vi "Instantiate.vi"(0 "location":string, 5 "insecurePort":string, 11 "error in (no error)":errorcluster) -> (4 "Measurement Client Wrapper out":refnum<class "Measurement Client Wrapper.lvclass">, 15 "error out":errorcluster)   [LabVIEW 2020, in "Measurement Client Wrapper.lvclass"]
uses:
  Measurement Client Wrapper.lvclass
  Measurement Client Wrapper.lvclass/Measurement Client Wrapper.ctl
  <vilib>/TAF/LabVIEW Measurement Client/Measurement_client-release.lvlib
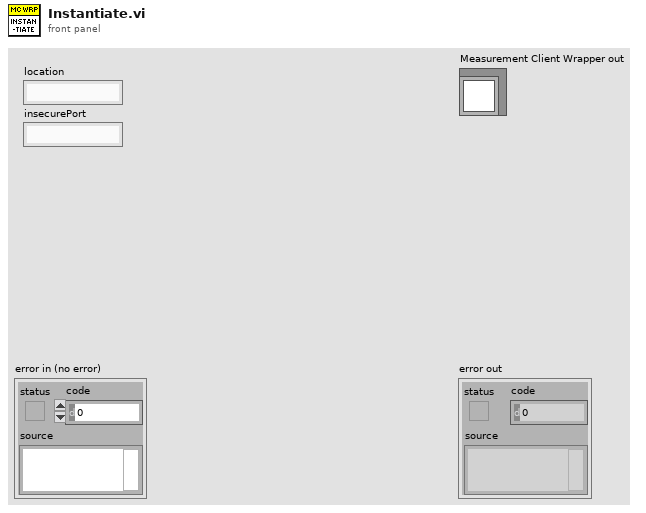
[diagram p1: front panel]
types:
  T1 = typedef "gprc-lvsupport-release.lvlib/grpcId.ctl" = u64
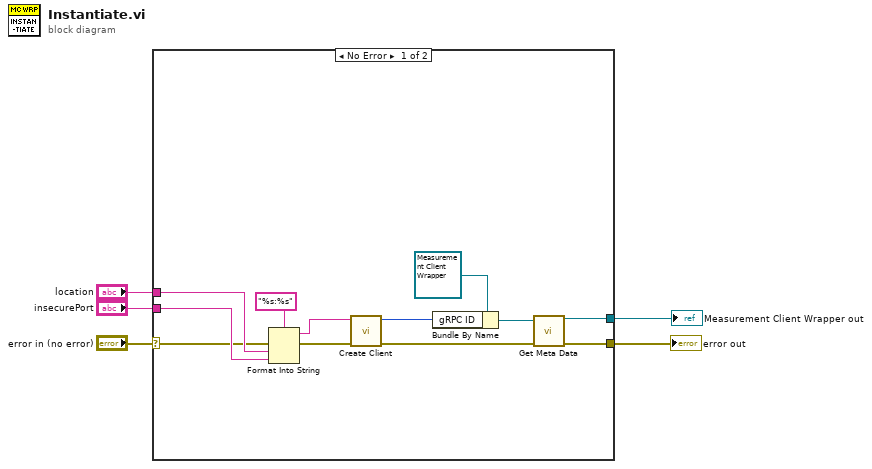
[diagram p0: block diagram]
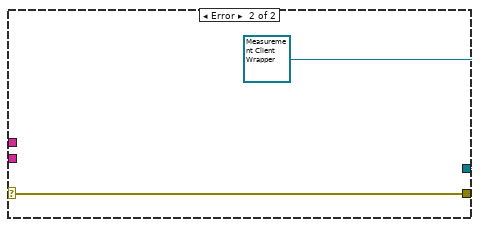
[diagram p2: hidden frame]
diagram:
  n1 = case shown="No Error" "error in (no error)" {
    selector: "error in (no error)" -> [w7 w19]
    tunnel: [w15 w19] -> w4
    tunnel: [w13 refnum<class "Measurement Client Wrapper.lvclass"> refnum ("Measurement Client Wrapper out")] -> w3
    tunnel: "location" -> [w10 _]
    tunnel: "insecurePort" -> [w9 _]
    frame No Error {
      n2 = Format Into String(format string="%s:%s", error in=w7, w10, w9) -> (resulting string=w8:string, error out=w6:errorcluster)  [unwired: 1 in]
      n3 = call <vilib>:"Create Client.vi"("error in"=w6, "address"=w8) -> ("error out"=w16:errorcluster, "gRPC ID Out"=w12:T1)  [unwired: 8 in]
      n4 = Bundle By Name(cluster=refnum<class "Measurement Client Wrapper.lvclass"> refnum ("Measurement Client Wrapper out"), "gRPC ID"=w12) -> (w14:refnum<class "Measurement Client Wrapper.lvclass">)
      n5 = call "Get Meta Data.vi"("Measurement Client Wrapper in"=w14, "error in"=w16) -> ("Measurement Client Wrapper out"=w13:refnum<class "Measurement Client Wrapper.lvclass">, "error out"=w15:errorcluster)  [unwired: 12 in]
    }
    frame Error {
    }
  }
  "error out" <- w4
  "Measurement Client Wrapper out" <- w3
